vi "Write_Single_Impedance_Meas.vi"(3 "Mean Signal\nImpedance cluster":T3, 4 "Current":waveform(dbl)[](array[waveform]), 5 "Run Impedances array":dbl[][](array[numeric]), 6 "Voltage":waveform(dbl)[](array[waveform]), 7 "Compensation and Gain":T1={"Rg_Vmon"=5000.0, "Rg_Imon"=5000.0, "ESL_Cal"=2.5e-07, "ESR_Cal"=0.0, "Cp_Cal"=0.0, "Rp_Cal"=0.0, "Use Open/Short\nCompensation"=FALSE, "R_Shunt"=10000.0}, 8 "Test Params Cluster":T2={"Test Freq. (Hz)"=0.0, "Output Signal Amplitude\nVolts Pk"=0.0, "Sampling Time (s)"=0.0, "Sampling Rate (Hz)"=0.0, "Output Channel"="Dev2/ao0", "Current Channel"="Dev2/ai0", "Voltage Channel"="Dev2/ai0", "Trigger Channel"="/Dev2/ao/StartTrigger", "Number of runs"=5}, 9 "Experiment Title":string="Experiment Title", 10 "File Name String":string="Test", 11 "Path":path=path "C:/Users/MPI/Documents/Test Saving Data") -> ()   [LabVIEW 2020]
panel:
  out "TDMS path":path=path "C:/Users/MPI/Documents/Test Saving Data/2022_01_06_23_07_06_Test.tdms"
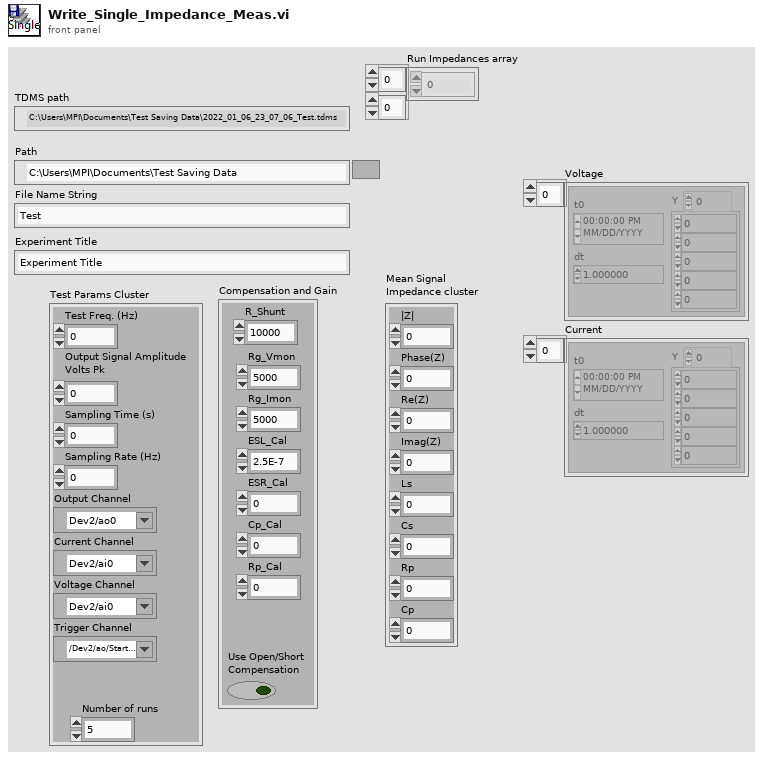
[diagram p1: front panel]
types:
  T1 = cluster{"Rg_Vmon":dbl, "Rg_Imon":dbl, "ESL_Cal":dbl, "ESR_Cal":dbl, "Cp_Cal":dbl, "Rp_Cal":dbl, "Use Open/Short\nCompensation":bool, "R_Shunt":dbl}
  T2 = cluster{"Test Freq. (Hz)":dbl, "Output Signal Amplitude\nVolts Pk":dbl, "Sampling Time (s)":dbl, "Sampling Rate (Hz)":dbl, "Output Channel":tag, "Current Channel":tag, "Voltage Channel":tag, "Trigger Channel":tag, "Number of runs":i32}
  T3 = cluster{"|Z|":dbl, "Phase(Z)":dbl, "Re(Z)":dbl, "Imag(Z)":dbl, "Ls":dbl, "Cs":dbl, "Rp":dbl, "Cp":dbl}
  T4 = enum16{"open", "open or create", "create or replace", "create", "open (read-only)"}
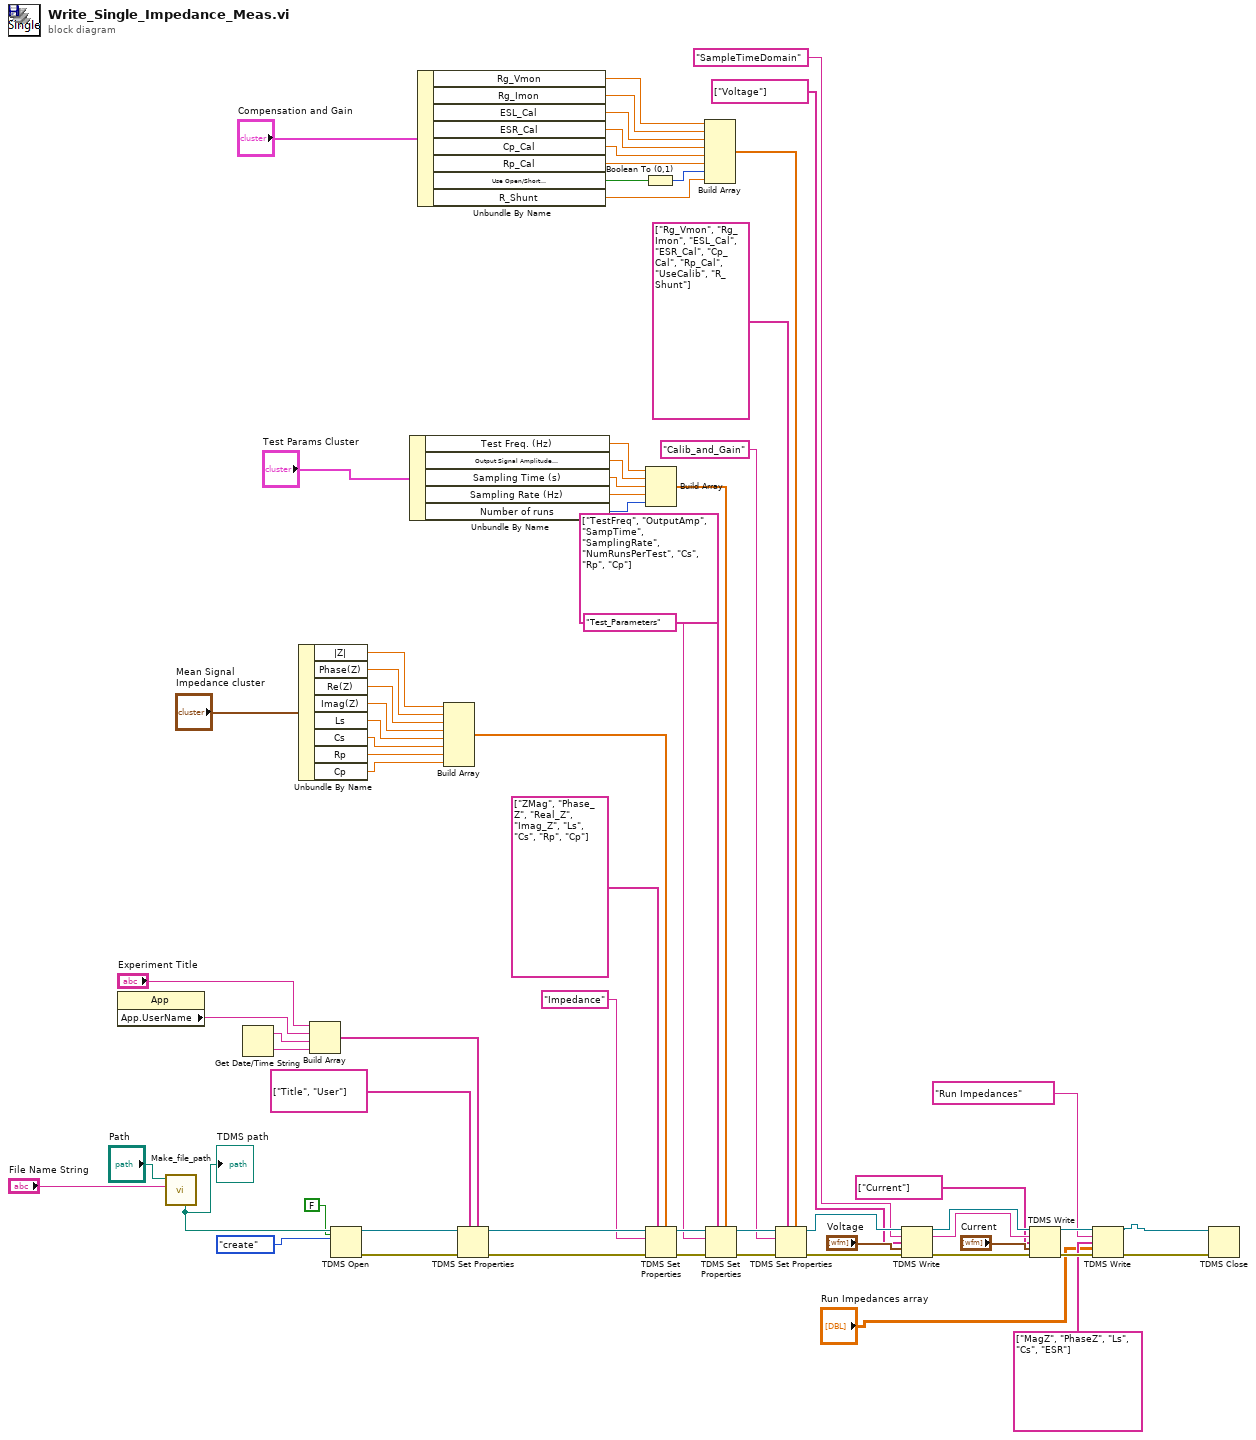
[diagram p0: block diagram]
diagram:
  n1 = property class="App"() -> ("App.UserName"=w64:string)  [unwired: 2 in, 2 out]
  n2 = call "Make_file_path.vi"("File Name String"="File Name String", "Base path"="Path") -> ("TDMS path"=w70:path)  [unwired: 9 in]
  "TDMS path" <- w70
  n3 = Get Date/Time String() -> (date string=w48:string, time string=w47:string)  [unwired: 3 in]
  n4 = Unbundle By Name("Mean Signal\nImpedance cluster") -> ("|Z|"=w57:dbl, "Phase(Z)"=w55:dbl, "Re(Z)"=w54:dbl, "Imag(Z)"=w53:dbl, "Ls"=w52:dbl, "Cs"=w51:dbl, "Rp"=w50:dbl, "Cp"=w49:dbl)
  n5 = Build Array("Experiment Title", w64, w48, w47) -> (w63:string[])
  n6 = TDMS Open(5:FALSE ("create index file? (T)"), 10:T4."create" ("operation (0:open)"), 11:w70) -> (0:w45:errorcluster, 3:w61:refnum<k34>)  [unwired: 4 in]
  n7 = Unbundle By Name("Test Params Cluster") -> ("Test Freq. (Hz)"=w36:dbl, "Output Signal Amplitude\nVolts Pk"=w37:dbl, "Sampling Time (s)"=w38:dbl, "Sampling Rate (Hz)"=w39:dbl, "Number of runs"=w1:i32)
  n8 = Unbundle By Name("Compensation and Gain") -> ("Rg_Vmon"=w28:dbl, "Rg_Imon"=w27:dbl, "ESL_Cal"=w26:dbl, "ESR_Cal"=w25:dbl, "Cp_Cal"=w24:dbl, "Rp_Cal"=w23:dbl, "Use Open/Short\nCompensation"=w22:bool, "R_Shunt"=w19:dbl)
  n9 = Build Array(w57, w55, w54, w53, w52, w51, w50, w49) -> (w58:dbl[])
  n10 = TDMS Set Properties(5:w63, 7:string[] ["Title", "User"] ("property names"), 8:w45, 11:w61) -> (0:w46:errorcluster, 3:w60:refnum<k34>)  [unwired: 4 out]
  n11 = Boolean To (0,1)(Boolean=w22) -> (0, 1=w21:i16)
  n12 = Build Array(w36, w37, w38, w39, w1) -> (w35:dbl[])
  n13 = TDMS Set Properties(5:w58, 7:string[] ["ZMag", "Phase_Z", "Real_Z", "Imag_Z", "Ls", "Cs", "Rp", "Cp"] ("property names"), 8:w46, 10:"Impedance" ("group name"), 11:w60) -> (0:w41:errorcluster, 3:w42:refnum<k34>)  [unwired: 3 out]
  n14 = Build Array(w28, w27, w26, w25, w24, w23, w21, w19) -> (w20:dbl[])
  n15 = TDMS Set Properties(5:w35, 7:string[] ["TestFreq", "OutputAmp", "SampTime", "SamplingRate", "NumRunsPerTest", "Cs", "Rp", "Cp"] ("property names"), 8:w41, 10:"Test_Parameters" ("group name"), 11:w42) -> (0:w31:errorcluster, 3:w32:refnum<k34>)  [unwired: 3 out]
  n16 = TDMS Set Properties(5:w20, 7:string[] ["Rg_Vmon", "Rg_Imon", "ESL_Cal", "ESR_Cal", "Cp_Cal", "Rp_Cal", "UseCalib", "R_Shunt"] ("property names"), 8:w31, 10:"Calib_and_Gain" ("group name"), 11:w32) -> (0:w15:errorcluster, 3:w18:refnum<k34>)  [unwired: 3 out]
  n17 = TDMS Write(0:w18, 5:"SampleTimeDomain" ("group name in (Untitled)"), 7:string[] ["Voltage"] ("channel name(s) in (Untitled)"), 9:"Voltage", 11:w15) -> (4:w17:refnum<k34>, 6:w11:string, 15:w16:errorcluster)  [unwired: 1 in, 1 out]
  n18 = TDMS Write(0:w17, 5:w11, 7:string[] ["Current"] ("channel name(s) in (Untitled)"), 9:"Current", 11:w16) -> (4:w5:refnum<k34>, 15:w6:errorcluster)  [unwired: 1 in, 2 out]
  n19 = TDMS Write(0:w5, 5:"Run Impedances" ("group name in (Untitled)"), 7:string[] ["MagZ", "PhaseZ", "Ls", "Cs", "ESR"] ("channel name(s) in (Untitled)"), 9:"Run Impedances array", 11:w6) -> (4:w8:refnum<k34>, 15:w7:errorcluster)  [unwired: 1 in, 2 out]
  n20 = TDMS Close(8:w7, 11:w8) -> ()  [unwired: 2 out]
